vi "Add Column.vi"(8 "error in (no error)":errorcluster, 11 "DataGrid Config Dialog in":refnum<class "DataGrid Config Dialog.lvclass">) -> (0 "error out":errorcluster, 3 "DataGrid Config Dialog out":refnum<class "DataGrid Config Dialog.lvclass">)   [LabVIEW 2018, in "DataGrid Config Dialog.lvclass"]
uses:
  DataGrid Config Dialog.lvclass
  DataGrid Config Dialog.lvclass/DataGrid Config Dialog.ctl
  Data Type Classes/Generic/Generic Data Type.lvclass
  DataGrid Config/Edit Configuration Actions.ctl
  Data Type Classes/Generic/Generic Data Type.lvclass/Generic Data Type.ctl
  Data Type Classes/Generic/Write Column Index.vi
  DataGrid Config/DataGrid Config.lvclass
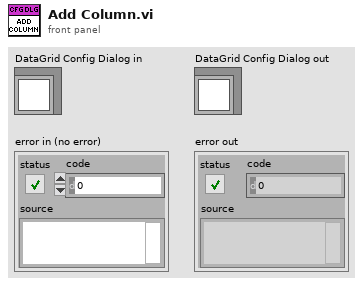
[diagram p1: front panel]
types:
  T1 = enum8{"Enabled", "Disabled", "Disabled and Grayed Out"}
  T2 = typedef "DataGrid Config.lvclass/Edit Configuration Actions.ctl" = enum16{"Add", "Remove", "Update", "Move Up", "Move Down"}
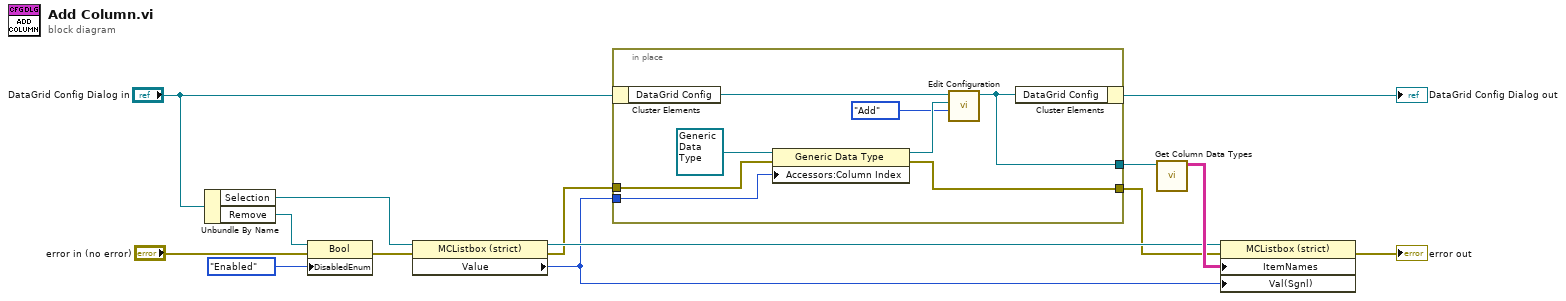
[diagram p0: block diagram]
diagram:
  n1 = Unbundle By Name("DataGrid Config Dialog in") -> ("Selection"=w12:refnum<vi>, "Remove"=w8:refnum<vi>)
  n2 = property class="Bool"(reference=w8, error in="error in (no error)", "DisabledEnum"=T1."Enabled" ("Disabled")) -> (error out=w5:errorcluster)  [unwired: 1 out]
  n3 = property class="MCListbox (strict)"(reference=w12, error in=w5) -> (reference out=w4:refnum<vi>, error out=w3:errorcluster, "Value"=w1:i32)
  n4 = in-place {
    in-place-border: [w18] -> w6
    in-place-border: w3 -> [w20]
    in-place-border: [w17] -> w2
    in-place-border: w1 -> [w19]
    n5 = in-place-cluster #1("DataGrid Config Dialog in") -> ("DataGrid Config"=w22:refnum<class "DataGrid Config.lvclass">)
    n6 = property class="Generic Data Type"(reference=refnum<class "Generic Data Type.lvclass"> refnum ("Generic Data Type"), error in=w20, "Accessors:Column Index"=w19) -> (reference out=w16:refnum<class "Generic Data Type.lvclass">, error out=w17:errorcluster)
    n7 = call "Edit Configuration.vi"("Edit Configuration Actions"=Edit_Configuration_Actions."Add", "Data Type Object"=w16, "DataGrid Config in"=w22) -> ("DataGrid Config out"=w18:refnum<class "DataGrid Config.lvclass">)  [unwired: 7 in, 1 out]
    n8 = in-place-cluster #1("DataGrid Config"=w18) -> (→"DataGrid Config Dialog out":refnum<class "DataGrid Config Dialog.lvclass">)
  }
  n9 = call "Get Column Data Types.vi"("DataGrid Config"=w6) -> ("Column Data Type Names"=w9:string[][])  [unwired: 10 in]
  n10 = property class="MCListbox (strict)"(reference=w4, error in=w2, "ItemNames"=w9, "Val(Sgnl)"=w1) -> (error out=→"error out":errorcluster)  [unwired: 1 out]
